vi "全局 时间2.vi"() -> ()   [LabVIEW 2016, in "数据传输系统.lvlib"]
panel:
  in  "浊度集成干预索引起始时间":string
  in  "水温集成干预索引起始时间":string
  in  "比电导率集成干预索引起始时间":string
  in  "PH集成干预索引起始时间":string
  in  "DO集成干预索引起始时间":string
  in  "CODCr集成干预索引起始时间":string
  in  "CODMn集成干预索引起始时间":string
  in  "总氮集成干预索引起始时间":string
  in  "总磷集成干预索引起始时间":string
  in  "氨氮集成干预索引起始时间":string
  in  "CODCr平行样索引起始时间":string
  in  "CODMn平行样索引起始时间":string
  in  "总氮平行样索引起始时间":string
  in  "总磷平行样索引起始时间":string
  in  "氨氮平行样索引起始时间":string
  in  "CODCr跨度核查索引起始时间":string
  in  "CODMn跨度核查索引起始时间":string
  in  "总氮跨度核查索引起始时间":string
  in  "总磷跨度核查索引起始时间":string
  in  "氨氮跨度核查索引起始时间":string
  in  "CODCr零点核查索引起始时间":string
  in  "CODMn零点核查索引起始时间":string
  in  "总氮零点核查索引起始时间":string
  in  "总磷零点核查索引起始时间":string
  in  "氨氮零点核查索引起始时间":string
  in  "标样核查索引起始时间":string
  in  "平行样索引起始时间":string
  in  "零点核查索引起始时间":string
  in  "跨度核查索引起始时间":string
  in  "加标回收索引起始时间":string
  in  "小时数据固定时间戳":string
  in  "小时数据时间2":string
  in  "时间2":string
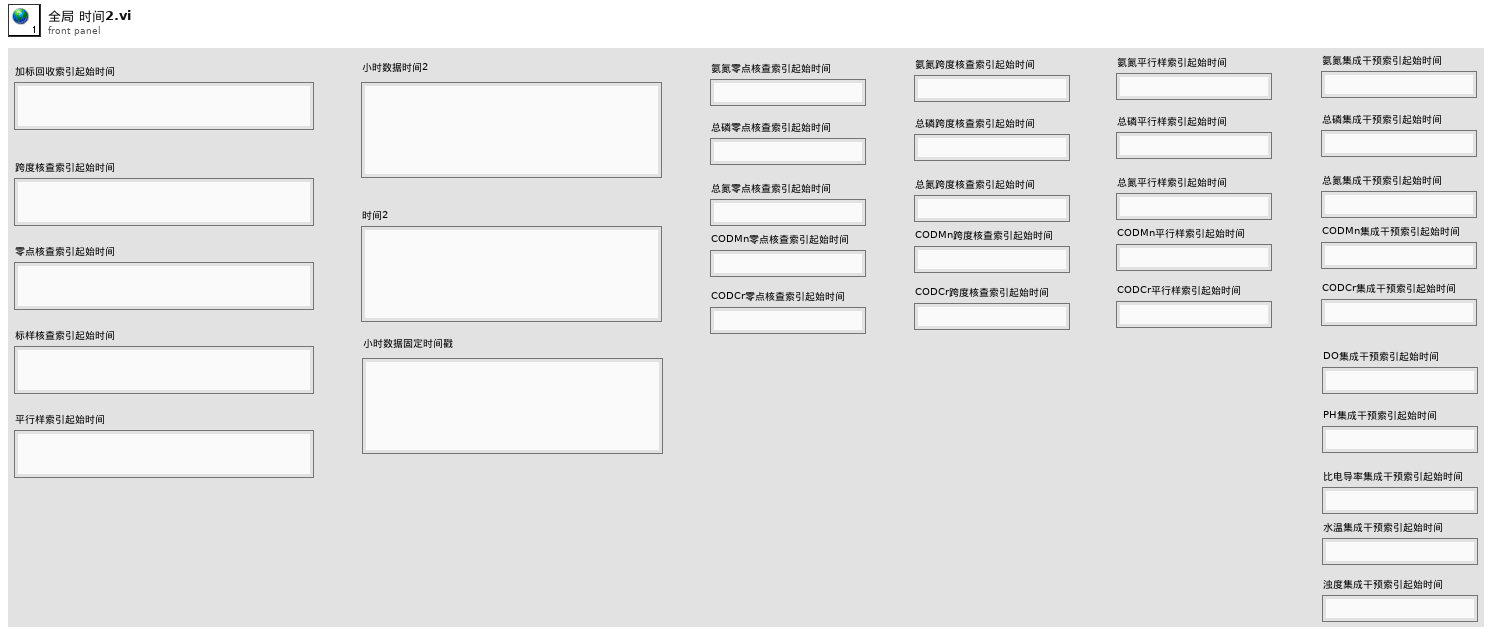
[diagram p1: front panel]
diagram:
